vi "Pos PID Controller.vi"(0 "Vel-Coefficient":dbl, 1 "Tolerance(deg)":dbl=0.5, 3 "Output Range(deg/s)":cluster{"output high":dbl, "output low":dbl}={"output high"=720.0, "output low"=-720.0} {"output low" format="%.2f"; "output high" format="%.2f"}, 5 "Reduction Ratio":dbl=1.0, 7 "Delta Motor Pos(deg)":dbl, 9 "Pos Passed(deg)":dbl, 11 "error in (no error)":errorcluster, 12 "Loop Time(ms)":u32=10, 14 "PID gains":T1={"proportional gain (Kc)"=6.5, "integral time (Ti, min)"=0.0075, "derivative time (Td, min)"=0.0005} {"derivative time (Td, min)" format="%.4f"; "integral time (Ti, min)" format="%.4f"; "proportional gain (Kc)" format="%.4f"}) -> (4 "Set Point(deg)":dbl=10.0, 6 "Output Vel(deg/s)":dbl format="%.2f", 10 "Process Var(deg)":dbl, 15 "error out":errorcluster)   [LabVIEW 2013, in "SGDV_Ctrl_v13_lib.lvlib"]
uses:
  SGDV_Ctrl_v13_lib.lvlib
  <vilib>/addons/control/pid/pid.llb/PID (DBL).vi
  <vilib>/addons/control/pid/NI_PID_pid.lvlib
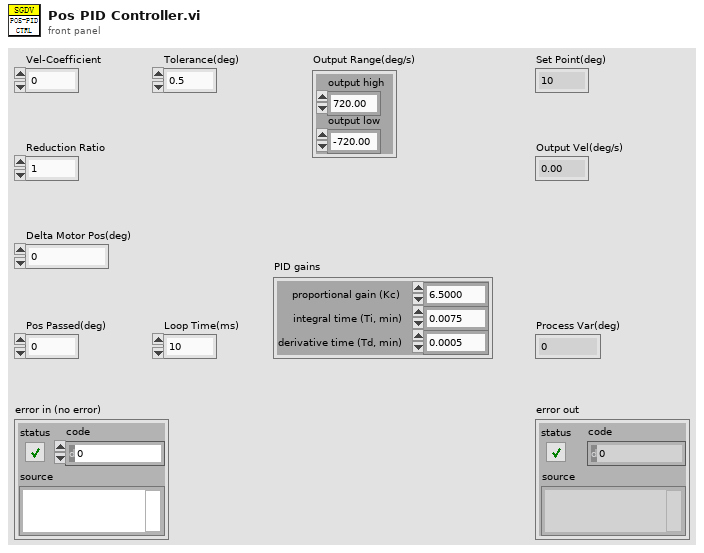
[diagram p1: front panel]
types:
  T1 = cluster{"proportional gain (Kc)":dbl, "integral time (Ti, min)":dbl, "derivative time (Td, min)":dbl}
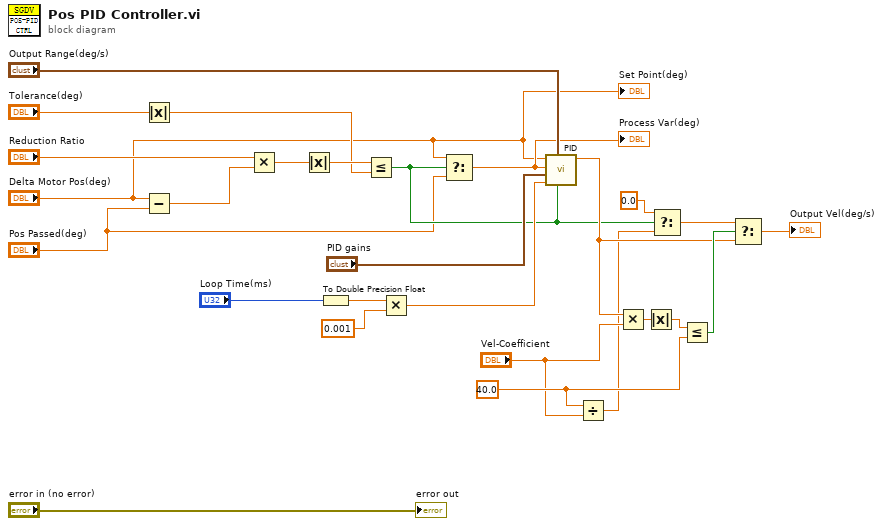
[diagram p0: block diagram]
diagram:
  w9 = 40.0 ("y")
  n1 = Absolute Value(x="Tolerance(deg)") -> (abs(x)=w20:dbl)
  n2 = Subtract(x="Delta Motor Pos(deg)", y="Pos Passed(deg)") -> (x-y=w3:dbl)
  n3 = Multiply(x="Reduction Ratio", y=w3) -> (x*y=w23:dbl)
  n4 = Absolute Value(x=w23) -> (abs(x)=w22:dbl)
  n5 = To Double Precision Float(number="Loop Time(ms)") -> (double precision float=w26:dbl)
  n6 = Less Or Equal?(x=w22, y=w20) -> (x <= y?=w11:bool)
  n7 = Multiply(x=w26, y=0.001) -> (x*y=w17:dbl)
  n8 = Select(t="Delta Motor Pos(deg)", s=w11, f="Pos Passed(deg)") -> (s? t:f=w16:dbl)
  "Process Var(deg)" <- w16
  n9 = call-poly <vilib>:"PID.vi"("reinitialize? (F)"=w11, "output range"="Output Range(deg/s)", "dt (s)"=w17, "PID gains"="PID gains", "process variable"=w16, "setpoint"="Delta Motor Pos(deg)") -> ("output"=w12:dbl)  [unwired: 4 in, 1 out]
  n10 = Divide(x=w9, y="Vel-Coefficient") -> (x/y=w7:dbl)
  n11 = Multiply(x=w12, y="Vel-Coefficient") -> (x*y=w14:dbl)
  n12 = Absolute Value(x=w14) -> (abs(x)=w13:dbl)
  n13 = Select(t=0.0 ("y"), s=w11, f=w7) -> (s? t:f=w6:dbl)
  n14 = Less Or Equal?(x=w13, y=w9) -> (x <= y?=w15:bool)
  n15 = Select(t=w6, s=w15, f=w12) -> (s? t:f=→"Output Vel(deg/s)":dbl)
  "Set Point(deg)" <- "Delta Motor Pos(deg)"
  "error out" <- "error in (no error)"
